vi "Result_Test.vi"(8 "error in (no error)":errorcluster caption="entrée d'erreur (pas d'erreur)", 11 "Flash_Jlink en entrée":refnum<class "Nodon_NI_Voltage_Channel_Check.lvclass">) -> (0 "error out":errorcluster caption="sortie d'erreur", 3 "Flash_Jlink en sortie":refnum<class "Nodon_NI_Voltage_Channel_Check.lvclass">)   [LabVIEW 2020, in "Library Test.lvlib" / "Nodon_NI_Voltage_Channel_Check.lvclass"]
uses:
  Nodon_NI_Voltage_Channel_Check.lvclass
  C:/Users/ngarcin/OneDrive - Altyor/Standard TB/Suite TB45/Class/Test/Test (Default)/Test (Default).lvclass
  Commun VI/TypeDef/Variable Printable.ctl
  <vilib>/measure/mascope.llb/Amplitude and Levels 1 chan.vi
  Test_Without_Instr/Test_Without_Inst.lvclass
  Commun VI/Library Commun.lvlib
  <vilib>/measure/NI_MAPro.lvlib
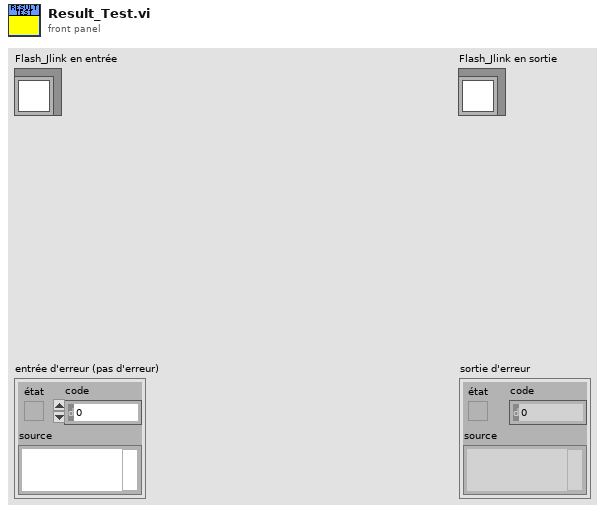
[diagram p1: front panel]
types:
  T1 = typedef "Variable Printable.ctl" = string
  T2 = enum16{"Get Variable", "Get All Variables", "Set Variable", "Delete Variable", "Delete All Variable"}
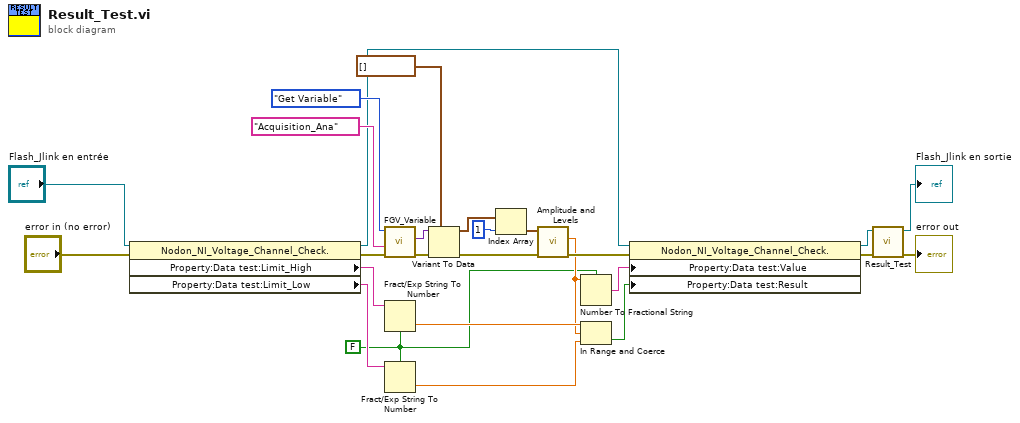
[diagram p0: block diagram]
diagram:
  w1 = FALSE ("utiliser le séparateur décimal du système (V)")
  n1 = property class="Nodon_NI_Voltage_Channel_Check."(reference="Flash_Jlink en entrée", error in="error in (no error)") -> (reference out=w14:refnum<class "Nodon_NI_Voltage_Channel_Check.lvclass">, error out=w16:errorcluster, "Property:Data test:Limit_High"=w8:string, "Property:Data test:Limit_Low"=w7:string)
  n2 = call "FGV_Variable.vi"("error in (no error)"=w16, "Variable"=T1 "Acquisition_Ana", "Function"=T2."Get Variable") -> ("error out"=w20:errorcluster, "Data Out"=w19:variant)  [unwired: 6 in, 1 out]
  n3 = Fract/Exp String To Number(use system decimal point (T)=w1, string=w8) -> (number=w5:dbl)  [unwired: 2 in, 1 out]
  n4 = Fract/Exp String To Number(use system decimal point (T)=w1, string=w7) -> (number=w6:dbl)  [unwired: 2 in, 1 out]
  n5 = Variant To Data(error in=w20, type=waveform(dbl)[] [] ("data"), Variant=w19) -> (data=w13:waveform(dbl)[], error out=w10:errorcluster)
  n6 = Index Array(array=w13, index=1 ("indice")) -> (element=w11:waveform(dbl))
  n7 = call-poly <vilib>:"Amplitude and Levels.vi"("error in (no error)"=w10, "signal in"=w11) -> ("error out"=w9:errorcluster, "high state level"=w3:dbl)  [unwired: 6 in, 2 out]
  n8 = Number To Fractional String(use system decimal point (T)=w1, number=w3) -> (F-format string=w2:string)  [unwired: 2 in]
  n9 = In Range and Coerce(upper limit=w5, x=w3, lower limit=w6) -> (In Range?=w4:bool)  [unwired: 1 out]
  n10 = property class="Nodon_NI_Voltage_Channel_Check."(reference=w14, error in=w9, "Property:Data test:Value"=w2, "Property:Data test:Result"=w4) -> (reference out=w23:refnum<class "Nodon_NI_Voltage_Channel_Check.lvclass">, error out=w24:errorcluster)
  n11 = call-parent "Result_Test.vi"("error in (no error)"=w24, "Test_Without_Inst en entrée"=w23) -> ("error out"=→"error out":errorcluster, "Test_Without_Inst en sortie"=→"Flash_Jlink en sortie":refnum<class "Nodon_NI_Voltage_Channel_Check.lvclass">)  [unwired: 8 in]
